vi "0 OCU.vi"(9 "Overview Image Ref In":T11, 10 "Map Name":T3="LPB Pool", 11 "Location of THINK":T14="127.0.0.1") -> ()   [LabVIEW 2011]
doc: "This is the current implementation of the operator control unit (OCU) for sailbot interfacing with this OCU over a network connection. The following features are currently implemented:\n- override control of the rudden angle and sail value by control interface or using keys\n- ability to add missions before and during a run, by clicking and by using GPS location of the boat or an auxiliary GPS attached to the OCU computer\n- modification of tuning values used on the boat\n- indicators for all relevant system status information\n\nAuthors: Jared Kirschner, Jason Curtis"
uses:
  2-Think/2 Typedefs/sail setpt.ctl
  2-Think/2 Typedefs/rudder angle.ctl
  2-Think/2 Typedefs/setpoints to boat.ctl
  0x2-OCU-Think Comm/0x2 Typedefs/manual override.ctl
  2-Think/2 Typedefs/eStopCommand.ctl
  0x2-OCU-Think Comm/0x2 Typedefs/Current Waypoint.ctl
  2-Think/2 Typedefs/UTM Location.ctl
  0x2-OCU-Think Comm/0x2 Classes/NetworkStreams/Reader/NetworkStreamReader.lvclass
  0x2-OCU-Think Comm/0x2 Classes/NetworkStreams/Reader/readType.ctl
  0x2-OCU-Think Comm/0x2 Typedefs/ocuMessage.ctl
  0x2-OCU-Think Comm/0x2 Typedefs/ocuCommands.ctl
  0x2-OCU-Think Comm/0x2 Classes/NetworkStreams/Writer/NetworkStreamWriter.lvclass
  2-Think/2 Typedefs/indicator LED.ctl
  2-Think/2 Typedefs/generalized sensor status.ctl
  2-Think/2 Typedefs/generalized actuator status.ctl
  2-Think/2 Typedefs/Which Boat.ctl
  2-Think/2 Typedefs/robot velocity.ctl
  2-Think/2 Typedefs/heading.ctl
  2-Think/2 Typedefs/rate of turn.ctl
  2-Think/2 Typedefs/pitch and roll.ctl
  2-Think/2 Typedefs/apparent wind.ctl
  2-Think/2 Typedefs/apparent wind speed.ctl
  2-Think/2 Typedefs/apparent wind direction.ctl
  2-Think/2 Typedefs/Velocity.ctl
  2-Think/2 Typedefs/absolute wind direction.ctl
  2-Think/2 Typedefs/absolute wind speed.ctl
  2-Think/2 Typedefs/absolute water current vector.ctl
  0x2-OCU-Think Comm/0x2 Typedefs/RIO-OCU update controls.ctl
  2-Think/2 Classes/Waypoint/Waypoint.lvclass
  0 Typedefs/Mission Type Radio Buttons.ctl
  2-Think/2 Classes/Missions/RoundBuoy/RoundBuoy.lvclass
  2-Think/2 Classes/Missions/PassBuoys/PassBuoys.lvclass
  2-Think/2 Classes/Missions/StationKeeping/StationKeeping.lvclass
  2-Think/2 Classes/Missions/Drive/DriveTo.lvclass
  2-Think/2 Typedefs/Goodness Fns Indicator.ctl
  2-Think/2 Typedefs/UTM Circle.ctl
  2-Think/2 Globals/2 Global.vi
  2-Think/2 Classes/Missions/GenericMission/GenericMission.lvclass
  2-Think/2 Typedefs/tacking attempt.ctl
  0 Typedefs/Sail Position.ctl
  0 Typedefs/Rudder Position.ctl
  0 Typedefs/Apparent Wind Point of Sail.ctl
  0x2-OCU-Think Comm/0x2 Typedefs/ocuWaypoint.ctl
  0x2-OCU-Think Comm/0x2 Typedefs/Waypoints List.ctl
  2-Think/2 Typedefs/PI Constants.ctl
  2-Think/2 Typedefs/Goodness Weightings.ctl
  0 Typedefs/Maps.ctl
  0 Typedefs/Location of Think.ctl
  <vilib>/vision/Image Controls.llb/IMAQ Image.ctl
  2-Think/2 Typedefs/Apparent Wind Mode.ctl
  0x2-OCU-Think Comm/0x2 Typedefs/Sail Setting Tuning.ctl
  0x2-OCU-Think Comm/0x2 Typedefs/Control values.ctl
panel:
  in  "Enable \nLocal GPS":bool
  out "Sensor Status":T1
  in  "GPS COM port":refnum<visa-resource-name>="COM1"
  in  "Additional inputs":T4(tab)
  in  "Manual Mission Input":enum32{"Drive", "Round", "Pass", "Station"}(tab)
  in  "Waypoint Location":enum32{"0", "1", "2", "3", "4"}(radio)
  in  "Buoy Side":enum32{"Starboard", "Port"}(radio)
  in  "Buoy to Round":enum32{"0", "1", "2", "3", "4"}(radio)
  in  "Starboard Buoy":enum32{"0", "1", "2", "3", "4"}(radio)=enum."1"
  in  "Port Buoy":enum32{"0", "1", "2", "3", "4"}(radio)
  in  "Buoy B":enum32{"0", "1", "2", "3", "4"}(radio)=enum."1"
  in  "Buoy A":enum32{"0", "1", "2", "3", "4"}(radio)
  in  "Add Mission":bool
  in  "Stored Locations Array":T5[](array[typedef])=[{"UTM Zone"=0.0, "Hemisphere"=enum."North", "East"=0.0, "North"=0.0}, {"UTM Zone"=0.0, "Hemisphere"=enum."North", "East"=0.0, "North"=0.0}, {"UTM Zone"=0.0, "Hemisphere"=enum."North", "East"=0.0, "North"=0.0}, {"UTM Zone"=0.0, "Hemisphere"=enum."North", "East"=0.0, "North"=0.0}, {"UTM Zone"=0.0, "Hemisphere"=enum."North", "East"=0.0, "North"=0.0}] {"North" format="%#_10f"; "East" format="%#_8f"}
  in  "Boat to Point 0":bool
  in  "Boat to Point 1":bool
  in  "Boat to Point 2":bool
  in  "Boat to Point 3":bool
  in  "Boat to Point 4":bool
  in  "Local to Point 4":bool
  in  "Local to Point 3":bool
  in  "Local to Point 2":bool
  in  "Local to Point 1":bool
  in  "Local to Point 0":bool
  in  "Update Constants":bool
  in  "Tuning Values":T6={"Goodness Weightings"={"Target Importance"=0.8, "No Sail Importance"=1.0, "Change Importance"=0.8, "Pure Waypoint \nImportance"=0.0, "Pure Wind \nImportance"=0.0}, "PI Constants"={"Proportional Gain"=0.5, "Integral Time"=0.0, "Derivative Time"=0.0}, "No Sail Zone\nTuning Quotient"=0.05, "Heading Change Wind Adjustment"=0.2, "Waypoint Tuning Quotient"=10.0, "Apparent Wind Mode"={"Desired Apparent\nWind Direction"=0.0, "On"=FALSE}, "Let Sail Out on Windcross"=TRUE, "Shift Goal for currents"=FALSE, "Round Buoy Safety"=5.0, "Sail Setting Options"={"Linear\nMode"=FALSE, "Sails Full In Point"=85.0, "Sails Full Out Point"=180.0}, "Defilter Wind Data"=TRUE, "Irons Range"=10.0, "Force tack attempt?"=FALSE, "Minimum\ntack try\ntime?"=35.0} {"Sail Setting Options"."Sails Full Out Point" step=0.1; "Sail Setting Options"."Sails Full In Point" step=0.1; "Apparent Wind Mode"."Desired Apparent\nWind Direction" step=0.1; "Goodness Weightings"."Pure Wind \nImportance" min=0.0 step=0.2; "Goodness Weightings"."Pure Waypoint \nImportance" min=0.0 step=0.2; "Goodness Weightings"."Change Importance" min=0.0 step=0.2; "Goodness Weightings"."No Sail Importance" min=0.0 step=0.2; "Goodness Weightings"."Target Importance" min=0.0 step=0.2}
  out "Battery Voltage":dbl
  out "Which Boat Am I?":T12
  out "Rudder Position":T13 scale=50.0..-50.0 scale format="%#.2g"
  out "Connected?":bool caption="Connection Status"
  in  "OVERRIDE SAIL?":bool
  in  "OVERRIDE RUDDER?":bool
  in  "Stop":bool
  in  "OCU Tab Control":enum32{"Mission [M]ap", "Detailed [T]elemetry"}(tab)
  in  "Map Mode":enum32{"M[i]ssion Edit", "M[o]nitoring"}(tab)
  in  "Load MDF":bool
  in  "Time(s)":dbl=300.0
  in  "Tolerance":dbl=3.0
  in  "Mission Entry Type":T15
  in  "Mission Def Filepath":path caption="MDF (Mission Definition File) path"
  in  "Reset Missions/Waypts":bool
  in  "Save Waypoints\nand PoI":bool
  out "Heading":T16 format="%05.1f"
  in  "Plot Colors":T17={"Target"=3381759, "No Sail"=16711680, "Change"=16756736, "Pure Waypt"=35080, "Pure Wind"=16860, "Combined"=16777228}
  out "Goodness Functions":picture
  out "Apparent Wind Direction\nPoint of Sail":T18 scale=0.0..360.0 scale format="%4d"
  out "Mission Status":string caption="Current Mission\nStatus"
  out "Tacking Attempt":T19
  in  "Log message":string caption="Log message (type and press enter)"
  in  "Save Image":bool
  out "Mission Map":T11(plugin-control)
  in  "Overlay Font Size":i16=40
  out "# of Waypts":i32
  in  "Globals":T20(tab)
  out "Don't Tip?":bool
  out "Wind Sensor Status":T1
  out "Estimated Error":dbl
  out "Robot Heading":T16 format="%05.1f"
  out "Robot UTM Location":T5 {"North" format="%#_10f"; "East" format="%#_8f"}
  out "Robot Velocity":T21
  out "Robot\nRate of Turn":T22 format="%05.1f"
  out "Robot Pitch/Roll":T23 {"Roll" format="%05.1f"; "Pitch" format="%05.1f"}
  out "Robot Speed (m/s)":dbl
  out "Absolute Wind":T24 {"East" format="%#_5g"}
  out "Apparent Wind Direction":T25
  out "Apparent Wind Speed":T26
  out "Apparent Wind":T27
  out "Crossing Wind":bool
  out "Setpoints to boat":T28
  out "Sail Position":T29
  out "Rudder Angle":T30
  out "Current Waypoint":T31
  in  "Reset to start":bool
  out "Manual Override":T32
  out "Waypoints Array":T33[](array[typedef]) {"UTM Location"."North" format="%#_10f"; "UTM Location"."East" format="%#_8f"}
  out "Waypoints Object Array":T34
  out "Mission Object Array":refnum<class "GenericMission.lvclass">[](array[class])
  out "Global No Sail Circles":T35[](array[typedef])
  out "Sail Position":T36
  # "PORT"
  # "STARB"
  # "Local GPS"
  # "Note: if THINK\nis on this computer,\nturning on local GPS will do strange things."
  # "HOWTO:\n1. save one or more points by moving GPS sensor to point, and pressing buttons below\n2. choose type of mission from tab control\n3. choose saved point(s) to load into mission. other params come from mission map input above\n4. click \"Add Mission\""
  # "P"
  # "S"
  # "O"
  # "O"
  # "A"
  # "B"
  # "HOWTO:\nchange values here, \nthen hit:"
  # "inputting missions:\nGo To Waypoint: set tolerance, and click on map.\nRound Buoy Port/Starboard: set tolerance, click.\nPass Between Buoys: Click one buoy location\nand drag to the other.\nStation Keeping: click southwest corner, drag to \nsoutheast corner. A square will be generated.\nTime(s) currently unimplemented.\nGlobal No-Sail Zone: click center of zone, drag to edge of\nzone. A circle with appropriate radius will be created."
  # "As Measured"
  # "Path Planning"
  # "From Planning Functions"
  # "(this is not a cluster because subitems\nare generated in parallel code)"
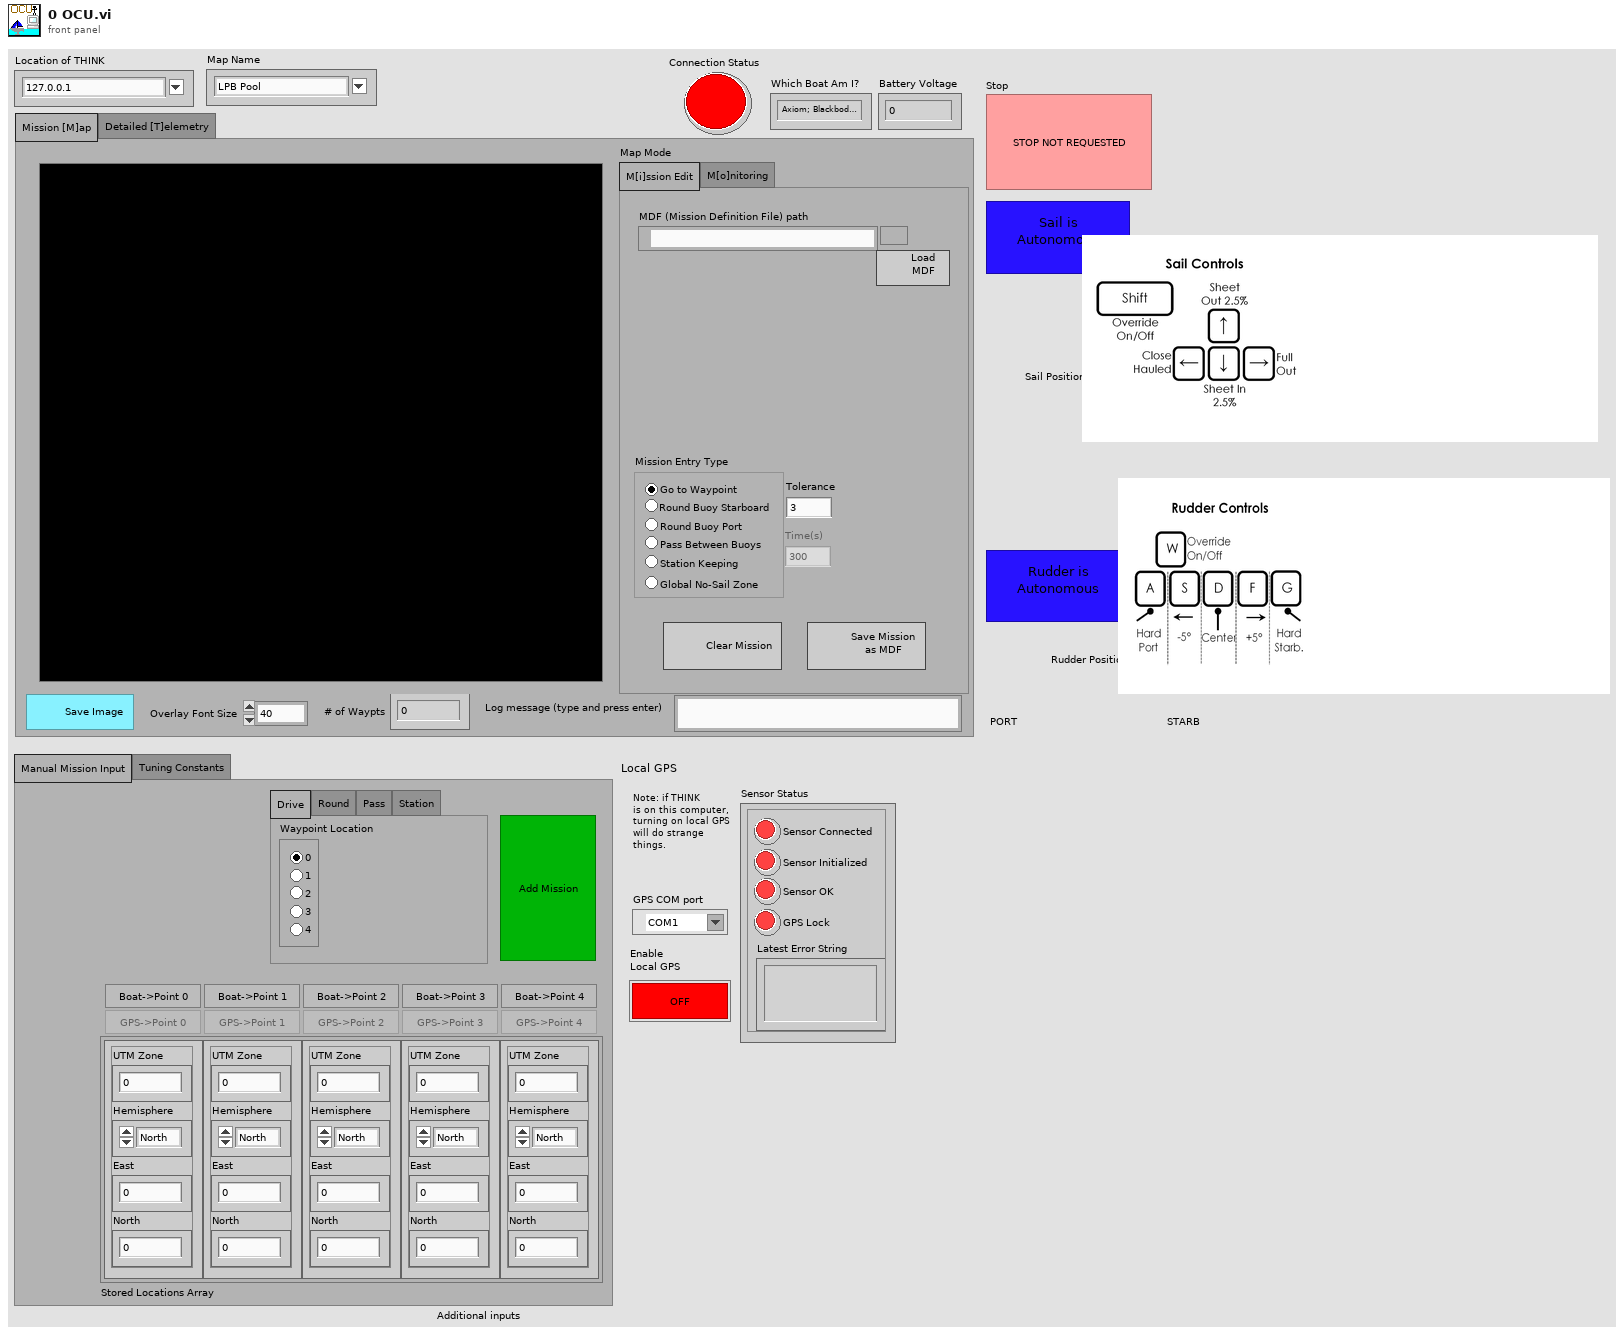
[diagram p1: front panel]
types:
  T1 = typedef "generalized sensor status.ctl" = cluster{"Sensor Connected":T2, "Sensor Initialized":T2, "Sensor OK":T2, "Latest Error String":string, "GPS Lock":T2}
  T2 = typedef "indicator LED.ctl" = bool
  T3 = typedef "Maps.ctl" = string
  T4 = enum32{"Manual Mission Input", "Tuning Constants"}
  T5 = typedef "UTM Location.ctl" = cluster{"UTM Zone":dbl, "Hemisphere":enum16{"North", "South"}, "East":dbl, "North":dbl}
  T6 = typedef "Control values.ctl" = cluster{"Goodness Weightings":T7, "PI Constants":T8, "No Sail Zone\nTuning Quotient":dbl, "Heading Change Wind Adjustment":dbl, "Waypoint Tuning Quotient":dbl, "Apparent Wind Mode":T9, "Let Sail Out on Windcross":bool, "Shift Goal for currents":bool, "Round Buoy Safety":dbl, "Sail Setting Options":T10, "Defilter Wind Data":bool, "Irons Range":dbl, "Force tack attempt?":bool, "Minimum\ntack try\ntime?":dbl}
  T7 = typedef "Goodness Weightings.ctl" = cluster{"Target Importance":dbl, "No Sail Importance":dbl, "Change Importance":dbl, "Pure Waypoint \nImportance":dbl, "Pure Wind \nImportance":dbl}
  T8 = typedef "PI Constants.ctl" = cluster{"Proportional Gain":dbl, "Integral Time":dbl, "Derivative Time":dbl}
  T9 = typedef "Apparent Wind Mode.ctl" = cluster{"Desired Apparent\nWind Direction":dbl, "On":bool}
  T10 = typedef "Sail Setting Tuning.ctl" = cluster{"Linear\nMode":bool, "Sails Full In Point":dbl, "Sails Full Out Point":dbl}
  T11 = typedef "IMAQ Image.ctl" = refnum<image>
  T12 = typedef "Which Boat.ctl" = enum16{"Axiom; Blackbody Radiation", "Simulation"}
  T13 = typedef "Rudder Position.ctl" = dbl
  T14 = typedef "Location of Think.ctl" = string
  T15 = typedef "Mission Type Radio Buttons.ctl" = enum32{"Go to Waypoint", "Round Buoy Starboard", "Round Buoy Port", "Pass Between Buoys", "Station Keeping", "Global No-Sail Zone"}
  T16 = typedef "heading.ctl" = dbl
  T17 = cluster{"Target":u32, "No Sail":u32, "Change":u32, "Pure Waypt":u32, "Pure Wind":u32, "Combined":u32}
  T18 = typedef "Apparent Wind Point of Sail.ctl" = dbl
  T19 = typedef "tacking attempt.ctl" = cluster{"attempting tack":bool, "tacking attempt\ntime remaining":dbl}
  T20 = enum32{"How Am I", "Where Am I", "What's Around Me", "Path Planning"}
  T21 = typedef "robot velocity.ctl" = cluster{"East":dbl, "North":dbl}
  T22 = typedef "rate of turn.ctl" = dbl
  T23 = typedef "pitch and roll.ctl" = cluster{"Pitch":dbl, "Roll":dbl}
  T24 = typedef "Velocity.ctl" = cluster{"East":dbl, "North":dbl}
  T25 = typedef "apparent wind direction.ctl" = dbl
  T26 = typedef "apparent wind speed.ctl" = dbl
  T27 = typedef "apparent wind.ctl" = cluster{"Toward Fore":dbl, "Toward Starboard":dbl}
  T28 = typedef "setpoints to boat.ctl" = cluster{"Sail Position":T29, "Rudder Angle":T30}
  T29 = typedef "sail setpt.ctl" = dbl
  T30 = typedef "rudder angle.ctl" = dbl
  T31 = typedef "Current Waypoint.ctl" = i32
  T32 = typedef "manual override.ctl" = cluster{"Override Active Rudder":bool, "Setpoints":T28, "Override Active Sail":bool}
  T33 = typedef "ocuWaypoint.ctl" = cluster{"Tolerance (m)":dbl, "UTM Location":T5}
  T34 = typedef "Waypoints List.ctl" = refnum<class "Waypoint.lvclass">[]
  T35 = typedef "UTM Circle.ctl" = cluster{"UTM Zone":dbl, "Hemisphere":enum16{"North", "South"}, "East":dbl, "North":dbl, "Radius":dbl}
  T36 = typedef "Sail Position.ctl" = dbl
  T37 = typedef "RIO-OCU update controls.ctl" = cluster{"Sensor Status":T1, "Battery Voltage":dbl, "Rudder Actuator Status":T38, "Sail Actuator Status":T38, "Which Boat Am I?":T12, "Robot Velocity":T21, "Robot UTM Location":T5, "Robot\nHeading ":T16, "Robot\nRate of Turn":T22, "Robot Pitch/Roll":T23, "Apparent Wind":T27, "Apparent Wind\nSpeed":T26, "Apparent Wind\nDirection (º)":T25, "Absolute Wind":T24, "Absolute Wind\nDirection (º)":T39, "Absolute Wind\nSpeed":T40, "Absolute Water Current Vector":T41, "Rudder Angle":T30, "Sail Position":T29, "Manual Override Cluster":T32, "Setpoints to boat":T28, "Current Waypoint":T31, "Think freq.":dbl, "Sense freq.":dbl, "Act freq.":dbl, "E-stop freq.":dbl, "Network \nfreq.":dbl, "Network \nLoop Iterations":i64, "E-Stop":bool, "Serialized Waypoint Array":string, "Serialized Mission Queue Elements":string, "Goodness Functions":T42, "Global No Sail Circles":T35[], "Optimal Heading":dbl, "Crossing Wind":bool, "Estimated Error":dbl, "Don't Tip?":bool, "Tacking Attempt":T19}
  T38 = typedef "generalized actuator status.ctl" = cluster{"Actuator Connected":T2}
  T39 = typedef "absolute wind direction.ctl" = dbl
  T40 = typedef "absolute wind speed.ctl" = dbl
  T41 = typedef "absolute water current vector.ctl" = cluster{"Direction":T25, "Magnitude":T25}
  T42 = typedef "Goodness Fns Indicator.ctl" = cluster{dbl, dbl, dbl[][]}
  T43 = typedef "0-Image Descriptor.ctl" = cluster{"Upper-Left Corner Coordinates":T5, "Meters/Pixel":dbl}
  T44 = typedef "NetworkStreamReader.lvclass/readType.ctl" = enum16{"Next in buffer", "Most current"}
  T45 = typedef "eStopCommand.ctl" = enum16{"Reset E-Stop", "Get E-Stop", "Set E-Stop"}
  T46 = cluster{"Image Ref Out":T11, "Image Descriptor":T43}
  T47 = typedef "ocuMessage.ctl" = cluster{"OCU Command":T48, "Data":variant}
  T48 = typedef "ocuCommands.ctl" = enum16{"Pass", "Send override", "Set waypoint number", "Stop", "Add Mission", "Reset Missions/Waypts", "Edit Control Values", "Add Global No-Sail", "Log Message"}
  T49 = enum8{"Enabled", "Disabled", "Disabled and Grayed Out"}
  T50 = typedef "eventvkey.ctl" = enum16{"ASCII", "Enter", "Return", "Shift", "Ctrl", "Alt", "Cmd", "Opt", "Caps", "NumLock", "Clear", "Break", "Up", "Down", "Left", "Right", "Insert", "Delete", "Home", "End", "PageUp", "PageDown", "Escape", "Help", "Pause", "ScrollLock", "F1", "F2", "F3", "F4", "F5", "F6", "F7", "F8", "F9", "F10", "F11", "F12", "F13", "F14", "F15", "F16", "F17", "F18", "F19", "F20", "F21", "F22", "F23", "F24", "Play", "VolumeUp", "VolumeDown", "Mute", "Two Byte Char"}
  T51 = cluster{"Global Rectangle":i32[], "Contours":cluster{"Contour Type":u32, "ROI Type":u32, "Points":i32[]}[]}
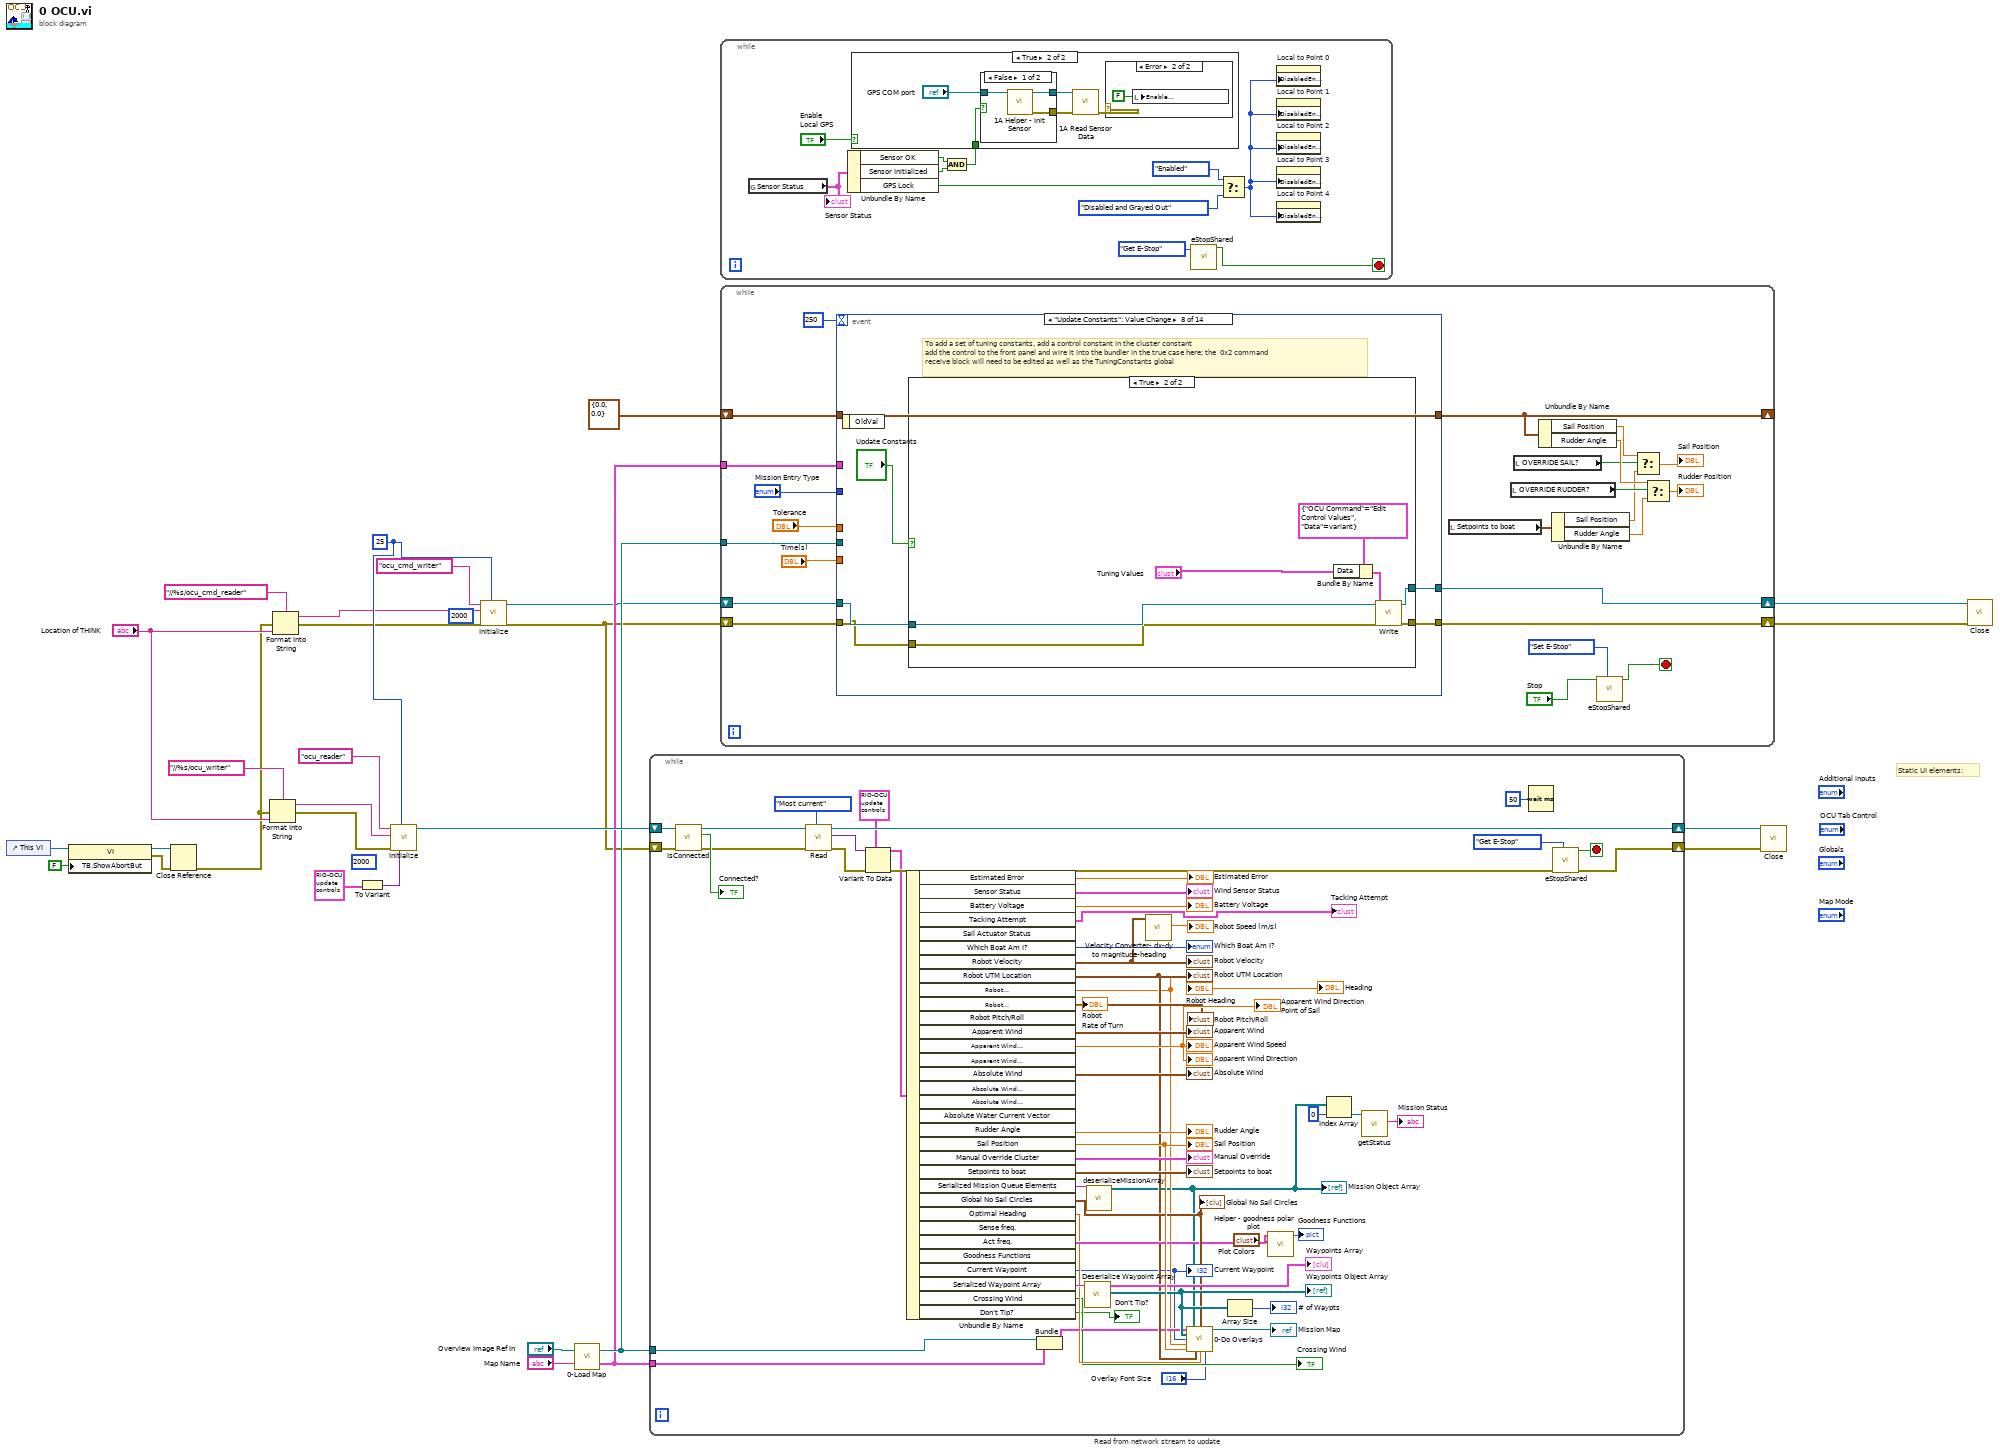
[diagram p0: block diagram]
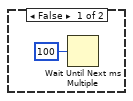
[diagram p2: hidden frame]
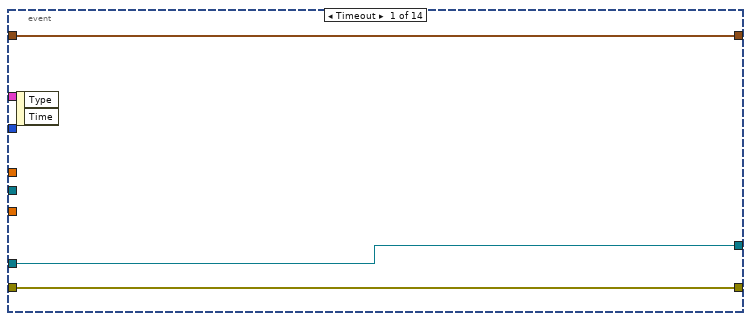
[diagram p5: hidden frame]
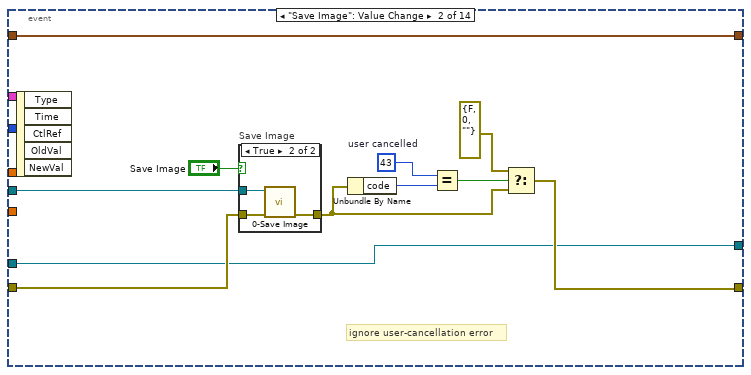
[diagram p6: hidden frame]
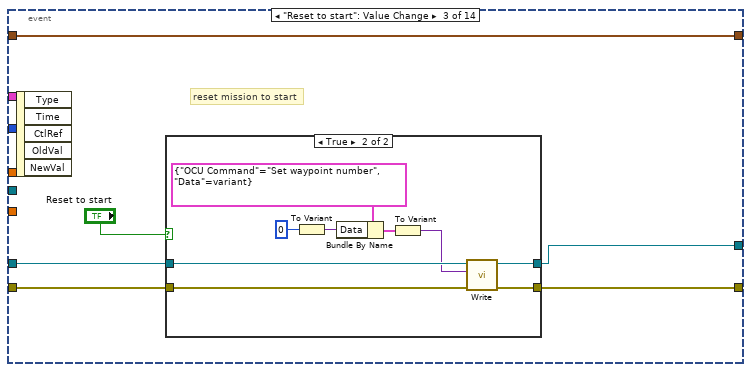
[diagram p8: hidden frame]
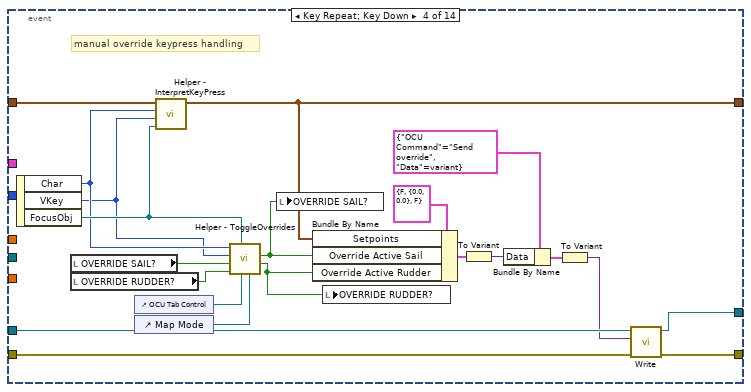
[diagram p10: hidden frame]
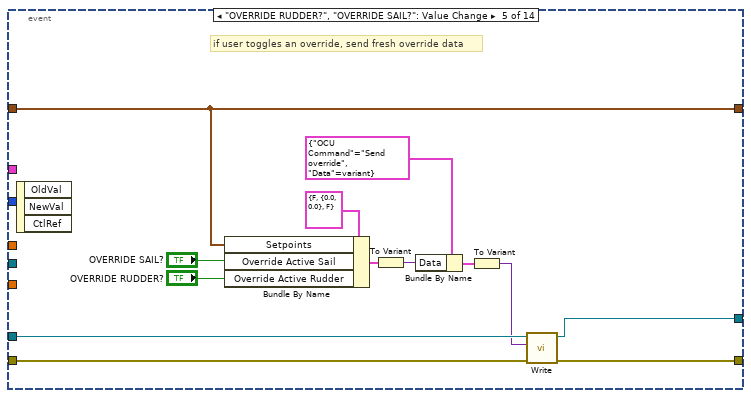
[diagram p11: hidden frame]
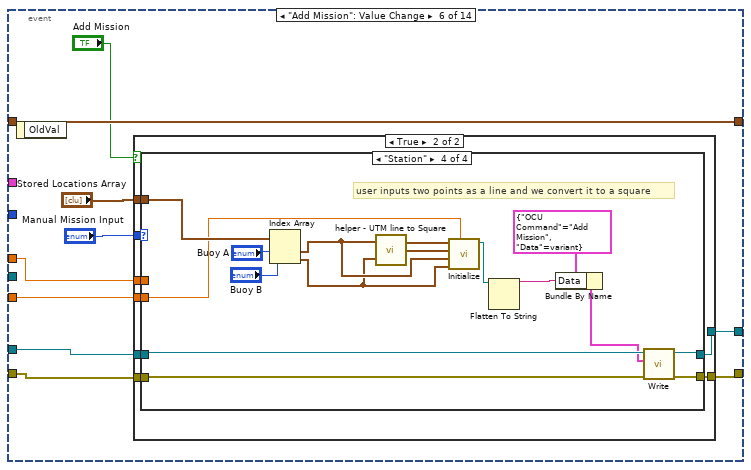
[diagram p12: hidden frame]
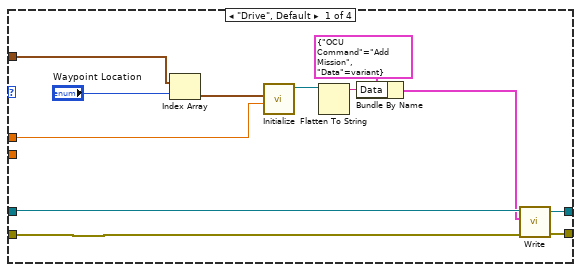
[diagram p14: hidden frame]
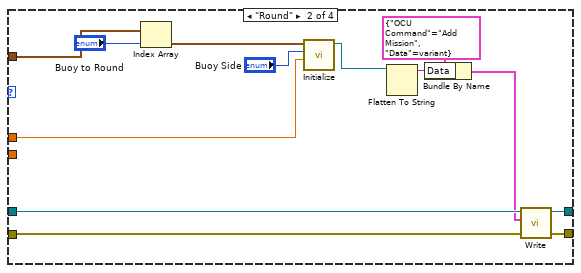
[diagram p15: hidden frame]
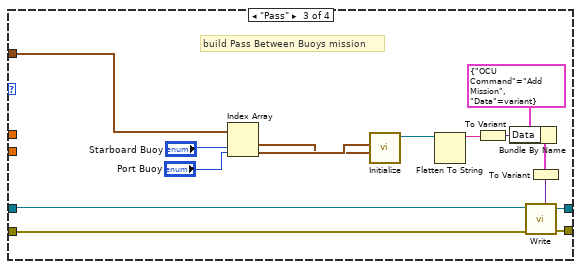
[diagram p16: hidden frame]
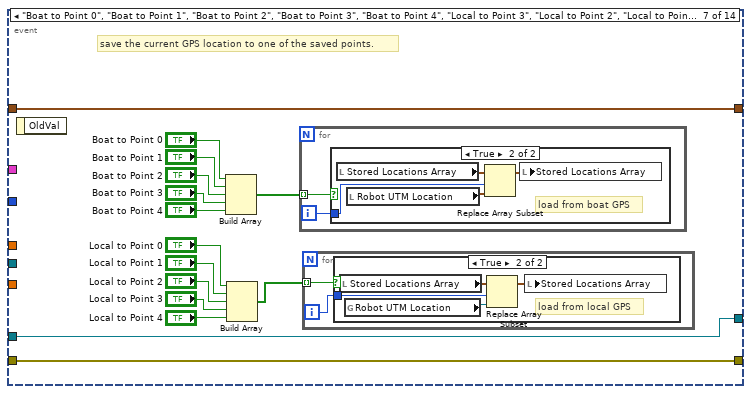
[diagram p17: hidden frame]
diagram:
  (unwired) 2000 ("connection timeout")
  (unwired) 2000 ("connection timeout")
  w27 = 25 ("writer buffer size")
  # "Static UI elements:"
  n1 = control-ref of="This VI"() -> (w17:refnum<vi>)
  n2 = property class="VI"(reference=w17, "TB.ShowAbortBut"=FALSE ("Tool Bar:Show Abort Button")) -> (reference out=w15:refnum<vi>, error out=w14:errorcluster)  [unwired: 1 in]
  n3 = Close Reference(reference=w15, error in (no error)=w14) -> (error out=w13:errorcluster)
  n4 = Format Into String(format string="//%s/ocu_writer", error in=w13, "Location of THINK") -> (resulting string=w7:string, error out=w11:errorcluster)  [unwired: 1 in]
  n5 = Format Into String(format string="//%s/ocu_cmd_reader", error in=w13, "Location of THINK") -> (resulting string=w5:string, error out=w12:errorcluster)  [unwired: 1 in]
  n6 = To Variant(anything=T37 {"Sensor Status"={"Sensor Connected"=FALSE, "Sensor Initialized"=FALSE, "Sensor OK"=FALSE, "Latest Error String"="", "GPS Lock"=FALSE}, "Battery Voltage"=0.0, "Rudder Actuator Status"={"Actuator Connected"=FALSE}, "Sail Actuator Status"={"Actuator Connected"=FALSE}, "Which Boat Am I?"=enum."Axiom; Blackbody Radiation", "Robot Velocity"={"East"=0.0, "North"=0.0}, "Robot UTM Location"={"UTM Zone"=0.0, "Hemisphere"=enum."North", "East"=0.0, "North"=0.0}, "Robot\nHeading "=0.0, "Robot\nRate of Turn"=0.0, "Robot Pitch/Roll"={"Pitch"=0.0, "Roll"=0.0}, "Apparent Wind"={"Toward Fore"=0.0, "Toward Starboard"=0.0}, "Apparent Wind\nSpeed"=0.0, "Apparent Wind\nDirection (º)"=0.0, "Absolute Wind"={"East"=0.0, "North"=0.0}, "Absolute Wind\nDirection (º)"=0.0, "Absolute Wind\nSpeed"=0.0, "Absolute Water Current Vector"={"Direction"=0.0, "Magnitude"=0.0}, "Rudder Angle"=0.0, "Sail Position"=0.0, "Manual Override Cluster"={"Override Active Rudder"=FALSE, "Setpoints"={"Sail Position"=0.0, "Rudder Angle"=0.0}, "Override Active Sail"=FALSE}, "Setpoints to boat"={"Sail Position"=0.0, "Rudder Angle"=0.0}, "Current Waypoint"=0, "Think freq."=0.0, "Sense freq."=0.0, "Act freq."=0.0, "E-stop freq."=0.0, "Network \nfreq."=0.0, "Network \nLoop Iterations"=0, "E-Stop"=FALSE, "Serialized Waypoint Array"="", "Serialized Mission Queue Elements"="", "Goodness Functions"={0.0, 0.0, []}, "Global No Sail Circles"=[], "Optimal Heading"=0.0, "Crossing Wind"=FALSE, "Estimated Error"=0.0, "Don't Tip?"=FALSE, "Tacking Attempt"={"attempting tack"=FALSE, "tacking attempt\ntime remaining"=0.0}} ("RIO->OCU update data")) -> (Variant=w26:variant)
  n7 = call "Initialize.vi"("Default return"=w26, "reader buffer size"=w27, "error in (no error)"=w11, "writer url"=w7, "reader name"="ocu_reader" ("writer name")) -> ("NetworkStreamWriter out"=w28:refnum<class "NetworkStreamReader.lvclass">)  [unwired: 5 in, 1 out]
  n8 = call "Initialize.vi"("writer buffer size"=w27, "error in (no error)"=w12, "reader url"=w5, "writer name"="ocu_cmd_writer") -> ("error out"=w1:errorcluster, "NetworkStreamWriter out"=w2:refnum<class "NetworkStreamWriter.lvclass">)  [unwired: 6 in]
  n9 = call "0-Load Map.vi"("Map Name"="Map Name", "Image Ref In"="Overview Image Ref In") -> ("Image Descriptor"=w9:T43, "Image Ref Out"=w23:T11)
  n10 = while "Read from network stream to update" {
    shift-right: [w86] -> w25
    shift-left: w28 -> [w81]
    shift-right: [w79] -> w24
    shift-left: w1 -> [w80]
    tunnel: w23 -> [w83]
    tunnel: w9 -> [w82]
    stop <- w84 stop-if-true
    n11 = call "IsConnected.vi"("error in (no error)"=w80, "NetworkStreamReader in"=w81) -> ("error out"=w75:errorcluster, "Connected?"=→"Connected?":bool, "NetworkStreamReader out"=w76:refnum<class "NetworkStreamReader.lvclass">)  [unwired: 7 in]
    n12 = call "Read.vi"("Read Type"=readType."Most current", "error in (no error)"=w75, "NetworkStreamReader in"=w76) -> ("error out"=w72:errorcluster, "element"=w71:variant, "NetworkStreamReader out"=w86:refnum<class "NetworkStreamReader.lvclass">)  [unwired: 4 in, 2 out]
    n13 = Variant To Data(error in=w72, type=T37 {"Sensor Status"={"Sensor Connected"=FALSE, "Sensor Initialized"=FALSE, "Sensor OK"=FALSE, "Latest Error String"="", "GPS Lock"=FALSE}, "Battery Voltage"=0.0, "Rudder Actuator Status"={"Actuator Connected"=FALSE}, "Sail Actuator Status"={"Actuator Connected"=FALSE}, "Which Boat Am I?"=enum."Axiom; Blackbody Radiation", "Robot Velocity"={"East"=0.0, "North"=0.0}, "Robot UTM Location"={"UTM Zone"=0.0, "Hemisphere"=enum."North", "East"=0.0, "North"=0.0}, "Robot\nHeading "=0.0, "Robot\nRate of Turn"=0.0, "Robot Pitch/Roll"={"Pitch"=0.0, "Roll"=0.0}, "Apparent Wind"={"Toward Fore"=0.0, "Toward Starboard"=0.0}, "Apparent Wind\nSpeed"=0.0, "Apparent Wind\nDirection (º)"=0.0, "Absolute Wind"={"East"=0.0, "North"=0.0}, "Absolute Wind\nDirection (º)"=0.0, "Absolute Wind\nSpeed"=0.0, "Absolute Water Current Vector"={"Direction"=0.0, "Magnitude"=0.0}, "Rudder Angle"=0.0, "Sail Position"=0.0, "Manual Override Cluster"={"Override Active Rudder"=FALSE, "Setpoints"={"Sail Position"=0.0, "Rudder Angle"=0.0}, "Override Active Sail"=FALSE}, "Setpoints to boat"={"Sail Position"=0.0, "Rudder Angle"=0.0}, "Current Waypoint"=0, "Think freq."=0.0, "Sense freq."=0.0, "Act freq."=0.0, "E-stop freq."=0.0, "Network \nfreq."=0.0, "Network \nLoop Iterations"=0, "E-Stop"=FALSE, "Serialized Waypoint Array"="", "Serialized Mission Queue Elements"="", "Goodness Functions"={0.0, 0.0, []}, "Global No Sail Circles"=[], "Optimal Heading"=0.0, "Crossing Wind"=FALSE, "Estimated Error"=0.0, "Don't Tip?"=FALSE, "Tacking Attempt"={"attempting tack"=FALSE, "tacking attempt\ntime remaining"=0.0}} ("RIO->OCU update data"), Variant=w71) -> (data=w69:T37, error out=w74:errorcluster)
    n14 = Unbundle By Name(w69) -> ("Estimated Error"=→"Estimated Error":dbl, "Sensor Status"=→"Wind Sensor Status":T1, "Battery Voltage"=→"Battery Voltage":dbl, "Tacking Attempt"=→"Tacking Attempt":T19, "Which Boat Am I?"=→"Which Boat Am I?":T12, "Robot Velocity"=w33:T21, "Robot UTM Location"=w45:T5, "Robot\nHeading"=w41:T16, "Robot\nRate of Turn"=→"Robot\nRate of Turn":T22, "Robot Pitch/Roll"=→"Robot Pitch/Roll":T23, "Apparent Wind"=→"Apparent Wind":T27, "Apparent Wind\nSpeed"=→"Apparent Wind Speed":T26, "Apparent Wind\nDirection (º)"=→"Apparent Wind Direction" →"Apparent Wind Direction\nPoint of Sail":T25, "Absolute Wind"=→"Absolute Wind":T24, "Rudder Angle"=→"Rudder Angle":T30, "Sail Position"=w57:T29, "Manual Override Cluster"=→"Manual Override":T32, "Setpoints to boat"=→"Setpoints to boat":T28, "Serialized Mission Queue Elements"=w52:string, "Global No Sail Circles"=w49:T35[], "Optimal Heading"=w44:dbl, "Goodness Functions"=w48:T42, "Current Waypoint"=w35:T31, "Serialized Waypoint Array"=w56:string, "Crossing Wind"=→"Crossing Wind":bool, "Don't Tip?"=→"Don't Tip?":bool)  [unwired: 6 out]
    "Robot UTM Location" <- w45
    "Robot Heading" <- w41
    "Robot Velocity" <- w33
    "Sail Position" <- w57
    "Current Waypoint" <- w35
    "Global No Sail Circles" <- w49
    "Heading" <- w41
    n15 = Bundle("Image Ref Out"=w83, "Image Descriptor"=w82) -> (w43:T46)  [unwired: 1 in]
    n16 = call "Deserialize Waypoint Array.vi"("Serialized Waypoint Array"=w56) -> ("Waypoints Object Array"=w54:T34, "Waypoints Array"=→"Waypoints Array":T33[])  [unwired: 9 in]
    "Waypoints Object Array" <- w54
    n17 = call "deserializeMissionArray.vi"("Serialized Mission Array"=w52) -> ("Mission Object Array"=w36:refnum<class "GenericMission.lvclass">[])  [unwired: 9 in, 1 out]
    "Mission Object Array" <- w36
    n18 = call "Velocity Converter- dx-dy to magnitude-heading.vi"("Vector In"=w33) -> ("Magnitude Out"=→"Robot Speed (m/s)":dbl)  [unwired: 9 in, 1 out]
    n19 = call "0-Do Overlays.vi"("Image Reference\nand Descriptor"=w43, "Missions"=w36, "No Sail Circles"=w49, "Waypoints"=w54, "Current Waypoint #"=w35, "Heading"=w41, "Sail Position"=w57, "Robot UTM Location"=w45, "Optimal Heading"=w44, "Font Size"="Overlay Font Size") -> ("Image out"=→"Mission Map":T11)  [unwired: 5 in]
    n20 = Array Size(array=w54) -> (size(s)=→"# of Waypts":i32)
    n21 = call "Helper - goodness polar plot.vi"("Plot Colors"="Plot Colors", "Goodness Fns In"=w48) -> ("Goodness Functions Polar Plot"=→"Goodness Functions":picture)  [unwired: 9 in]
    n22 = Index Array(array=w36, index=0) -> (element=w37:refnum<class "GenericMission.lvclass">)
    n23 = call-dynamic "getStatus.vi"("GenericMission in"=w37) -> ("Status"=→"Mission Status":string)  [unwired: 8 in, 2 out]
    n24 = Wait (ms)(milliseconds to wait=u32 50 ("millisecond multiple")) -> ()  [unwired: 1 out]
    n25 = call "eStopShared.vi"("Command"=eStopCommand."Get E-Stop", "Error In"=w74) -> ("Error Out"=w79:errorcluster, "E-Stop Out"=w84:bool)  [unwired: 8 in]
  }
  n26 = while {
    shift-right: [w108] -> w18
    shift-left: w1 -> [w87]
    shift-right: [w102] -> _
    shift-left: T28 {"Sail Position"=0.0, "Rudder Angle"=0.0} ("Setpoints") -> [w110]
    shift-right: [w104] -> w19
    shift-left: w2 -> [w88]
    tunnel: w23 -> [w103]
    tunnel: w9 -> [w101]
    stop <- w107 stop-if-true
    n27 = event shown="[7] \"Update Constants\": Value Change" {
      selector: _ -> [_ _ _ _ _ _ _ _ _ _ _ _ _ _]
      dyn-events: _ -> [_ _ _ _ _ _ _ _ _ _ _ _ _ _]
      timeout: 250 -> [_ _ _ _ _ _ _ _ _ _ _ _ _ _]
      tunnel: w110 -> [w113 w120 w134 w166 w169 w187 w263 w287 w309 w325 w334 w375 w393 w513]
      tunnel: [w113 w120 w134 w164 w169 w187 w263 w287 w309 w325 w334 w375 w393 w513] -> w102
      tunnel: w87 -> [w111 w118 w131 w161 w176 w188 w261 w284 w301 w324 w332 w373 w392 w514]
      tunnel: [w111 w115 w129 w160 w175 w185 w261 w282 w299 w324 w331 w371 w390 w514] -> w108
      tunnel: w88 -> [w112 w114 w132 w163 w178 w189 w262 w285 w300 w323 w330 w374 w388 w515]
      tunnel: [w112 w114 w130 w162 w177 w184 w262 w283 w302 w323 w329 w372 w389 w515] -> w104
      tunnel: w103 -> [_ w119 _ _ _ _ _ _ _ _ _ _ _ _]
      tunnel: w101 -> [_ _ _ _ _ _ _ _ _ _ _ _ w391 _]
      tunnel: "Mission Entry Type" -> [_ _ _ _ _ _ _ _ _ _ _ _ w387 _]
      tunnel: "Tolerance" -> [_ _ _ _ _ w186 _ _ _ _ _ _ w386 _]
      tunnel: "Time(s)" -> [_ _ _ _ _ w180 _ _ _ _ _ _ w385 _]
      event Timeout {
        n28 = event-data() -> ()  [unwired: 1 in, 2 out]
      }
      event "Save Image": Value Change {
        w123 = 43  # user cancelled
        # "ignore user-cancellation error"
        n29 = event-data() -> ()  [unwired: 1 in, 5 out]
        n30 = case "Save Image" shown="True" "Save Image" {
          tunnel: w118 -> [w125 w128]
          tunnel: [w125 w127] -> w117
          tunnel: w119 -> [_ w126]
          frame False {
          }
          frame True {
            n31 = call "0-Save Image.vi"("Error In"=w128, "Image in"=w126) -> ("Error Out"=w127:errorcluster)  [unwired: 9 in]
          }
        }
        n32 = Unbundle By Name(w117) -> ("code"=w124:i32)
        n33 = Equal?(x=w123, y=w124) -> (x = y?=w122:bool)
        n34 = Select(t=errorcluster {"status"=FALSE, "code"=0, "source"=""}, s=w122, f=w117) -> (s? t:f=w115:errorcluster)
      }
      event "Reset to start": Value Change {
        # "reset mission to start"
        n35 = event-data() -> ()  [unwired: 1 in, 5 out]
        n36 = case shown="True" "Reset to start" {
          tunnel: w132 -> [w136 w142]
          tunnel: w131 -> [w135 w143]
          tunnel: [w136 w145] -> w130
          tunnel: [w135 w144] -> w129
          frame False {
          }
          frame True {
            n37 = To Variant(anything=T31 0 ("Current Waypoint")) -> (Variant=w140:variant)
            n38 = Bundle By Name(cluster=T47 {"OCU Command"=enum."Set waypoint number", "Data"=variant}, "Data"=w140) -> (w138:T47)
            n39 = To Variant(anything=w138) -> (Variant=w137:variant)
            n40 = call "Write.vi"("error in (no error)"=w143, "element"=w137, "NetworkStreamWriter in"=w142) -> ("error out"=w144:errorcluster, "NetworkStreamWriter out"=w145:refnum<class "NetworkStreamWriter.lvclass">)  [unwired: 7 in]
          }
        }
      }
      event Key Repeat; Key Down {
        # "manual override keypress handling"
        n41 = event-data() -> ("Char"=w153:i16, "VKey"=w152:T50, "FocusObj"=w154:refnum<vi>)  [unwired: 1 in]
        n42 = local read "OVERRIDE SAIL?"() -> (w151:bool)
        n43 = local read "OVERRIDE RUDDER?"() -> (w150:bool)
        n44 = control-ref of="OCU Tab Control"() -> (w147:refnum<vi>)
        n45 = control-ref of="Map Mode"() -> (w146:refnum<vi>)
        n46 = call "Helper - InterpretKeyPress.vi"("FocusObj"=w154, "VKey"=w152, "Char"=w153, "Command In"=w166) -> ("Command Out"=w164:T28)  [unwired: 7 in]
        n47 = call "Helper - ToggleOverrides.vi"("Map Mode Tab Control Ref"=w146, "OCU Tab Control Ref"=w147, "FocusObj"=w154, "Rudder Override?"=w150, "Sail Override?"=w151, "VKey"=w152, "Char"=w153) -> ("Override Rudder"=w149:bool, "Override Sail"=w148:bool)  [unwired: 3 in]
        n48 = local write "OVERRIDE SAIL?"(w148) -> ()
        n49 = Bundle By Name(cluster=T32 {"Override Active Rudder"=FALSE, "Setpoints"={"Sail Position"=0.0, "Rudder Angle"=0.0}, "Override Active Sail"=FALSE} ("Manual Override Cluster"), "Setpoints"=w164, "Override Active Sail"=w148, "Override Active Rudder"=w149) -> (w156:T32)
        n50 = local write "OVERRIDE RUDDER?"(w149) -> ()
        n51 = To Variant(anything=w156) -> (Variant=w159:variant)
        n52 = Bundle By Name(cluster=T47 {"OCU Command"=enum."Send override", "Data"=variant}, "Data"=w159) -> (w158:T47)
        n53 = To Variant(anything=w158) -> (Variant=w155:variant)
        n54 = call "Write.vi"("error in (no error)"=w161, "element"=w155, "NetworkStreamWriter in"=w163) -> ("error out"=w160:errorcluster, "NetworkStreamWriter out"=w162:refnum<class "NetworkStreamWriter.lvclass">)  [unwired: 7 in]
      }
      event "OVERRIDE RUDDER?", "OVERRIDE SAIL?": Value Change {
        # "if user toggles an override, send fresh override data"
        n55 = event-data() -> ()  [unwired: 1 in, 3 out]
        n56 = Bundle By Name(cluster=T32 {"Override Active Rudder"=FALSE, "Setpoints"={"Sail Position"=0.0, "Rudder Angle"=0.0}, "Override Active Sail"=FALSE} ("Manual Override Cluster"), "Setpoints"=w169, "Override Active Sail"="OVERRIDE SAIL?", "Override Active Rudder"="OVERRIDE RUDDER?") -> (w171:T32)
        n57 = To Variant(anything=w171) -> (Variant=w174:variant)
        n58 = Bundle By Name(cluster=T47 {"OCU Command"=enum."Send override", "Data"=variant}, "Data"=w174) -> (w173:T47)
        n59 = To Variant(anything=w173) -> (Variant=w170:variant)
        n60 = call "Write.vi"("error in (no error)"=w176, "element"=w170, "NetworkStreamWriter in"=w178) -> ("error out"=w175:errorcluster, "NetworkStreamWriter out"=w177:refnum<class "NetworkStreamWriter.lvclass">)  [unwired: 7 in]
      }
      event "Add Mission": Value Change {
        n61 = event-data() -> ()  [unwired: 1 in, 1 out]
        n62 = case shown="True" "Add Mission" {
          tunnel: w189 -> [w191 w199]
          tunnel: w188 -> [w190 w198]
          tunnel: w186 -> [_ w197]
          tunnel: [w190 w196] -> w185
          tunnel: [w191 w195] -> w184
          tunnel: "Manual Mission Input" -> [_ w194]
          tunnel: "Stored Locations Array" -> [_ w193]
          tunnel: w180 -> [_ w192]
          frame False {
          }
          frame True {
            n63 = case shown="\"Station\"" w194 {
              tunnel: w198 -> [w207 w220 w229 w247]
              tunnel: [w211 w220 w232 w252] -> w196
              tunnel: w197 -> [w208 w223 _ _]
              tunnel: [w210 w222 w233 w253] -> w195
              tunnel: w199 -> [w209 w221 w234 w251]
              tunnel: w193 -> [w202 w218 w228 w246]
              tunnel: w192 -> [_ _ _ w239]
              frame "Drive", Default {
                n64 = Index Array(array=w202, index="Waypoint Location") -> (element=w205:T5)
                n65 = call "Initialize.vi"("Tolerance (m)"=w208, "Drive Location"=w205) -> ("Drive out"=w203:refnum<class "DriveTo.lvclass">)  [unwired: 8 in, 1 out]
                n66 = Flatten To String(anything=w203) -> (data string=w201:string)  [unwired: 3 in, 2 out]
                n67 = Bundle By Name(cluster=T47 {"OCU Command"=enum."Add Mission", "Data"=variant}, "Data"=w201) -> (w200:T47)
                n68 = call "Write.vi"("error in (no error)"=w207, "element"=w200, "NetworkStreamWriter in"=w209) -> ("error out"=w211:errorcluster, "NetworkStreamWriter out"=w210:refnum<class "NetworkStreamWriter.lvclass">)  [unwired: 7 in]
              }
              frame "Round" {
                n69 = Index Array(array=w218, index="Buoy to Round") -> (element=w217:T5)
                n70 = call "Initialize.vi"("Tolerance (m)"=w223, "Round side?"="Buoy Side", "Buoy to Round"=w217) -> ("RoundBuoys out"=w212:refnum<class "RoundBuoy.lvclass">)  [unwired: 7 in, 1 out]
                n71 = Flatten To String(anything=w212) -> (data string=w214:string)  [unwired: 3 in, 2 out]
                n72 = Bundle By Name(cluster=T47 {"OCU Command"=enum."Add Mission", "Data"=variant}, "Data"=w214) -> (w213:T47)
                n73 = call "Write.vi"("element"=w213, "NetworkStreamWriter in"=w221) -> ("NetworkStreamWriter out"=w222:refnum<class "NetworkStreamWriter.lvclass">)  [unwired: 8 in, 1 out]
              }
              frame "Pass" {
                # "build Pass Between Buoys mission"
                n74 = Index Array(array=w228, index #1="Starboard Buoy", index #2="Port Buoy") -> (element #1=w224:T5, element #2=w225:T5)
                n75 = call "Initialize.vi"("Buoy Pass 2"=w224, "Buoy Pass 1"=w225) -> ("PassBuoys out"=w230:refnum<class "PassBuoys.lvclass">)  [unwired: 8 in, 1 out]
                n76 = Flatten To String(anything=w230) -> (data string=w236:string)  [unwired: 3 in, 2 out]
                n77 = To Variant(anything=w236) -> (Variant=w237:variant)
                n78 = Bundle By Name(cluster=T47 {"OCU Command"=enum."Add Mission", "Data"=variant}, "Data"=w237) -> (w235:T47)
                n79 = To Variant(anything=w235) -> (Variant=w231:variant)
                n80 = call "Write.vi"("error in (no error)"=w229, "element"=w231, "NetworkStreamWriter in"=w234) -> ("error out"=w232:errorcluster, "NetworkStreamWriter out"=w233:refnum<class "NetworkStreamWriter.lvclass">)  [unwired: 7 in]
              }
              frame "Station" {
                # "user inputs two points as a line and we convert it to a square"
                n81 = Index Array(array=w246, index #1="Buoy A", index #2="Buoy B") -> (element #1=w243:T5, element #2=w242:T5)
                n82 = call "helper - UTM line to Square.vi"("Endpoint 2, UTM"=w242, "Endpoint 1, UTM"=w243) -> ("Endpoint 4, UTM"=w249:T5, "Endpoint 3, UTM"=w248:T5)
                n83 = call "Initialize.vi"("Duration (s)"=w239, "Buoy SE"=w242, "Buoy SW"=w243, "Buoy NE"=w249, "Buoy NW"=w248) -> ("StationKeeping out"=w250:refnum<class "StationKeeping.lvclass">)  [unwired: 5 in, 1 out]
                n84 = Flatten To String(anything=w250) -> (data string=w241:string)  [unwired: 3 in, 2 out]
                n85 = Bundle By Name(cluster=T47 {"OCU Command"=enum."Add Mission", "Data"=variant}, "Data"=w241) -> (w240:T47)
                n86 = call "Write.vi"("error in (no error)"=w247, "element"=w240, "NetworkStreamWriter in"=w251) -> ("error out"=w252:errorcluster, "NetworkStreamWriter out"=w253:refnum<class "NetworkStreamWriter.lvclass">)  [unwired: 7 in]
              }
            }
          }
        }
      }
      event "Boat to Point 0", "Boat to Point 1", "Boat to Point 2", "Boat to Point 3", "Boat to Point 4", "Local to Point 3", "Local to Point 2", "Local to Point 1", "Local to Point 0", "Local to Point 4": Value Change {
        # "save the current GPS location to one of the saved points."
        n87 = event-data() -> ()  [unwired: 1 in, 1 out]
        n88 = Build Array("Boat to Point 0", "Boat to Point 1", "Boat to Point 2", "Boat to Point 3", "Boat to Point 4") -> (w264:bool[])
        n89 = Build Array("Local to Point 0", "Local to Point 1", "Local to Point 2", "Local to Point 3", "Local to Point 4") -> (w255:bool[])
        n90 = for {
          tunnel: w264 -> [w277] mode=indexing
          i -> [w276]
          n91 = case shown="True" w277 {
            tunnel: w276 -> [_ w279]
            frame False {
            }
            frame True {
              # "load from boat GPS"
              n92 = local read "Stored Locations Array"() -> (w281:T5[])
              n93 = local read "Robot UTM Location"() -> (w278:T5)
              n94 = Replace Array Subset(array=w281, new element=w278, index=w279) -> (w280:T5[])
              n95 = local write "Stored Locations Array"(w280) -> ()
            }
          }
        }
        n96 = for {
          tunnel: w255 -> [w271] mode=indexing
          i -> [w270]
          n97 = case shown="True" w271 {
            tunnel: w270 -> [_ w272]
            frame False {
            }
            frame True {
              # "load from local GPS"
              n98 = local read "Stored Locations Array"() -> (w274:T5[])
              n99 = global read "2 Global.vi" "Robot UTM Location"() -> (w273:refnum<class "UTM_Location.lvclass">)
              n100 = Replace Array Subset(array=w274, new element=w273, index=w272) -> (w275:T5[])
              n101 = local write "Stored Locations Array"(w275) -> ()
            }
          }
        }
      }
      event "Update Constants": Value Change {
        # "To add a set of tuning constants, add a control constant in the cluster constant\nadd the control to the front panel and wire it into the bundler in the true case here; the  0x2 command\nreceive block will need to be edited as well as the TuningConstants global"
        n102 = event-data() -> ()  [unwired: 1 in, 1 out]
        n103 = case shown="True" "Update Constants" {
          tunnel: w285 -> [w289 w295]
          tunnel: w284 -> [w288 w294]
          tunnel: [w289 w293] -> w283
          tunnel: [w288 w292] -> w282
          frame False {
          }
          frame True {
            n104 = Bundle By Name(cluster=T47 {"OCU Command"=enum."Edit Control Values", "Data"=variant}, "Data"="Tuning Values") -> (w291:T47)
            n105 = call "Write.vi"("error in (no error)"=w294, "element"=w291, "NetworkStreamWriter in"=w295) -> ("error out"=w292:errorcluster, "NetworkStreamWriter out"=w293:refnum<class "NetworkStreamWriter.lvclass">)  [unwired: 7 in]
          }
        }
      }
      event "Log message": Key Up {
        # "Remove carriage\nreturn."
        # "Enter key?"
        n106 = event-data() -> ("ScanCode"=w298:i16)  [unwired: 1 in, 2 out]
        n107 = Equal?(x=w298, y=i16 28) -> (x = y?=w307:bool)
        n108 = Search and Replace String(replace all?=TRUE ("replace all? (F)"), input string="Log message", search string="\n" ("string"), replace string="") -> (result string=w304:string)  [unwired: 4 in, 3 out]
        n109 = case "Was the log message entered?" shown="True" w307 {
          tunnel: [w311 w320] -> w302
          tunnel: [w310 w319] -> w299
          tunnel: w301 -> [w310 w314]
          tunnel: w300 -> [w311 w318]
          tunnel: w304 -> [_ w315]
          frame False {
          }
          frame True {
            n110 = To Variant(anything=w315) -> (Variant=w322:variant)
            n111 = property on="Log message" class="Str"(error in=w314, "Value"="") -> (error out=w313:errorcluster)  [unwired: 1 in, 1 out]
            n112 = Bundle By Name(cluster=T47 {"OCU Command"=enum."Log Message", "Data"=variant}, "Data"=w322) -> (w321:T47)
            n113 = To Variant(anything=w321) -> (Variant=w316:variant)
            n114 = call "Write.vi"("error in (no error)"=w313, "element"=w316, "NetworkStreamWriter in"=w318) -> ("error out"=w319:errorcluster, "NetworkStreamWriter out"=w320:refnum<class "NetworkStreamWriter.lvclass">)  [unwired: 7 in]
          }
        }
      }
      event "Save Waypoints\nand PoI": Value Change {
        n115 = event-data() -> ()  [unwired: 1 in, 1 out]
        n116 = case "Save MDF" shown="True" "Save Waypoints\nand PoI" {
          frame False {
          }
          frame True {
            n117 = local read "Global No Sail Circles"() -> (w327:T35[])
            n118 = local read "Mission Object Array"() -> (w328:refnum<class "GenericMission.lvclass">[])
            n119 = call "0-Write MDF.vi"("Global No Sail Circles"=w327, "Missions (Object Array)"=w328) -> ()  [unwired: 3 in, 1 out]
          }
        }
      }
      event "Load MDF": Value Change {
        n120 = event-data() -> ()  [unwired: 1 in, 1 out]
        n121 = case "Load MDF" shown="True" "Load MDF" {
          tunnel: w332 -> [w335 w338]
          tunnel: [w335 w345] -> w331
          tunnel: w330 -> [w336 w340]
          tunnel: [w336 w343] -> w329
          frame False {
          }
          frame True {
            w342 = T47 {"OCU Command"=enum."Reset Missions/Waypts", "Data"=variant}  # clear missions
            n122 = To Variant(anything=w342) -> (Variant=w341:variant)
            n123 = call "Write.vi"("error in (no error)"=w338, "element"=w341, "NetworkStreamWriter in"=w340) -> ("error out"=w337:errorcluster, "NetworkStreamWriter out"=w339:refnum<class "NetworkStreamWriter.lvclass">)  [unwired: 7 in]
            n124 = call "0-Read MDF.vi"("Error in"=w337, "MDF file path"="Mission Def Filepath") -> ("Error out"=w347:errorcluster, "Global No Sail Circles"=w349:T35[], "Missions (Object Array)"=w348:refnum<class "GenericMission.lvclass">[])  [unwired: 1 in]
            n125 = for {
              tunnel: w348 -> [w360] mode=indexing
              shift-right: [w366] -> w346
              shift-left: w347 -> [w362]
              shift-right: [w364] -> w344
              shift-left: w339 -> [w365]
              n126 = Flatten To String(anything=w360, error in (no error)=w362) -> (data string=w361:string, error out=w363:errorcluster)  [unwired: 2 in, 1 out]
              n127 = To Variant(anything=w361) -> (Variant=w368:variant)
              n128 = Bundle By Name(cluster=T47 {"OCU Command"=enum."Add Mission", "Data"=variant}, "Data"=w368) -> (w369:T47)
              n129 = To Variant(anything=w369) -> (Variant=w367:variant)
              n130 = call "Write.vi"("error in (no error)"=w363, "element"=w367, "NetworkStreamWriter in"=w365) -> ("error out"=w366:errorcluster, "NetworkStreamWriter out"=w364:refnum<class "NetworkStreamWriter.lvclass">)  [unwired: 7 in]
            }
            n131 = local write "Mission Object Array"(w348) -> ()
            n132 = local write "Global No Sail Circles"(w349) -> ()
            n133 = for {
              tunnel: w349 -> [w352] mode=indexing
              shift-right: [w355] -> w345
              shift-left: w346 -> [w351]
              shift-right: [w353] -> w343
              shift-left: w344 -> [w354]
              n134 = To Variant(anything=w352) -> (Variant=w357:variant)
              n135 = Bundle By Name(cluster=T47 {"OCU Command"=enum."Add Global No-Sail", "Data"=variant}, "Data"=w357) -> (w358:T47)
              n136 = To Variant(anything=w358) -> (Variant=w356:variant)
              n137 = call "Write.vi"("error in (no error)"=w351, "element"=w356, "NetworkStreamWriter in"=w354) -> ("error out"=w355:errorcluster, "NetworkStreamWriter out"=w353:refnum<class "NetworkStreamWriter.lvclass">)  [unwired: 7 in]
            }
          }
        }
      }
      event "Reset Missions/Waypts": Value Change {
        n138 = event-data() -> ()  [unwired: 1 in, 1 out]
        n139 = case "Reset Missions" shown="True" "Reset Missions/Waypts" {
          tunnel: w374 -> [w378 w384]
          tunnel: w373 -> [w377 w383]
          tunnel: [w378 w382] -> w372
          tunnel: [w377 w381] -> w371
          frame False {
          }
          frame True {
            n140 = To Variant(anything=T47 {"OCU Command"=enum."Reset Missions/Waypts", "Data"=variant}) -> (Variant=w379:variant)
            n141 = call "Write.vi"("error in (no error)"=w383, "element"=w379, "NetworkStreamWriter in"=w384) -> ("error out"=w381:errorcluster, "NetworkStreamWriter out"=w382:refnum<class "NetworkStreamWriter.lvclass">)  [unwired: 7 in]
          }
        }
      }
      event "Mission Map": Mouse Up {
        # "add a waypoint to the list"
        n142 = event-data() -> ()  [unwired: 1 in, 1 out]
        n143 = case shown="\"Global No-Sail Zone\"" w387 {
          selector: w387 -> [_ _ w467 _ _]
          tunnel: w392 -> [w403 w429 w474 w492 w512]
          tunnel: [w401 w439 w471 w483 w503] -> w390
          tunnel: w391 -> [w402 w426 w456 w478 w510]
          tunnel: w386 -> [w396 _ w468 _ w493]
          tunnel: [w399 w437 w460 w486 w504] -> w389
          tunnel: w388 -> [w398 w436 w457 w487 w502]
          tunnel: w385 -> [_ _ _ _ w494]
          frame "Go to Waypoint", Default {
            n144 = property on="Mission Map" class="ImageControl"(error in=w403) -> (error out=w405:errorcluster, "Last Mouse Position"=w404:cluster{"X":i32, "Y":i32})  [unwired: 1 in, 1 out]
            n145 = call "Helper - Image To UTM.vi"("Image Descriptor"=w402, "Pixel Coordinates"=w404) -> ("UTM Location"=w394:T5)  [unwired: 1 in, 1 out]
            n146 = invoke on="Mission Map" class="ImageControl" method="Clear ROI"(error in=w405) -> (error out=w400:errorcluster)  [unwired: 2 in, 2 out]
            n147 = disable-structure shown="Enabled" {
              disable-tunnel: w396 -> [w412 w415]
              disable-tunnel: [w408 w419] -> w395
              disable-tunnel: w394 -> [w406 w414]
              frame Enabled {
                n148 = call "Initialize.vi"("Tolerance (m)"=w412, "Drive Location"=w406) -> ("Drive out"=w407:refnum<class "DriveTo.lvclass">)  [unwired: 8 in, 1 out]
                n149 = Flatten To String(anything=w407) -> (data string=w409:string)  [unwired: 3 in, 2 out]
                n150 = To Variant(anything=w409) -> (Variant=w410:variant)
                n151 = Bundle By Name(cluster=T47 {"OCU Command"=enum."Add Mission", "Data"=variant}, "Data"=w410) -> (w408:T47)
              }
              frame Disabled {
                n152 = call "init_waypoint.vi"("Coords"=w414, "Tolerance (m)"=w415) -> ("Waypoint Out"=w413:refnum<class "Waypoint.lvclass">)  [unwired: 9 in]
                n153 = Flatten To String(anything=w413) -> (data string=w416:string)  [unwired: 3 in, 2 out]
                n154 = To Variant(anything=w416) -> (Variant=w417:variant)
                n155 = Bundle By Name(cluster=T47 {"OCU Command"=enum."Set waypoint number", "Data"=variant}, "Data"=w417) -> (w419:T47)
              }
            }
            n156 = To Variant(anything=w395) -> (Variant=w397:variant)
            n157 = call "Write.vi"("error in (no error)"=w400, "element"=w397, "NetworkStreamWriter in"=w398) -> ("error out"=w401:errorcluster, "NetworkStreamWriter out"=w399:refnum<class "NetworkStreamWriter.lvclass">)  [unwired: 7 in]
          }
          frame "Global No-Sail Zone" {
            n158 = property on="Mission Map" class="ImageControl"(error in=w429) -> (error out=w428:errorcluster, "ROI"=w430:T51)  [unwired: 1 in, 1 out]
            n159 = call "helper- line ROI to 2 UTM Pts.vi"("ROI"=w430, "Image Descriptor"=w426) -> ("Endpoint UTM 2"=w425:T5, "Endpoint UTM 1"=w427:T5)
            n160 = Unbundle By Name(w425) -> ("East"=w423:dbl, "North"=w424:dbl)
            n161 = Unbundle By Name(w427) -> ("UTM Zone"=w431:dbl, "Hemisphere"=w432:enum16{"North", "South"}, "East"=w421:dbl, "North"=w422:dbl)
            n162 = call "2 XYPointsToDistanceAndAngle.vi"("East 2"=w424, "North 2"=w423, "East 1"=w422, "North 1"=w421) -> ("Distance"=w420:dbl)  [unwired: 6 in, 1 out]
            n163 = invoke on="Mission Map" class="ImageControl" method="Clear ROI"(error in=w428) -> (error out=w438:errorcluster)  [unwired: 2 in, 2 out]
            n164 = disable-structure shown="Enabled" {
              disable-tunnel: w420 -> [w445 w451]
              disable-tunnel: [w447 w455] -> w434
              disable-tunnel: T35 {"UTM Zone"=0.0, "Hemisphere"=enum."North", "East"=0.0, "North"=0.0, "Radius"=0.0} ("UTM Location") -> [w446 _]
              disable-tunnel: w422 -> [w444 _]
              disable-tunnel: w421 -> [w443 _]
              disable-tunnel: w432 -> [w442 _]
              disable-tunnel: w431 -> [w441 _]
              frame Enabled {
                n165 = Bundle By Name(cluster=w446, "UTM Zone"=w441, "Hemisphere"=w442, "East"=w443, "North"=w444, "Radius"=w445) -> (w440:T35)
                n166 = To Variant(anything=w440) -> (Variant=w448:variant)
                n167 = Bundle By Name(cluster=T47 {"OCU Command"=enum."Add Global No-Sail", "Data"=variant}, "Data"=w448) -> (w447:T47)
              }
              frame Disabled {
                n168 = call "init_waypoint.vi"("Tolerance (m)"=w451) -> ("Waypoint Out"=w450:refnum<class "Waypoint.lvclass">)  [unwired: 10 in]
                n169 = Flatten To String(anything=w450) -> (data string=w452:string)  [unwired: 3 in, 2 out]
                n170 = To Variant(anything=w452) -> (Variant=w453:variant)
                n171 = Bundle By Name(cluster=T47 {"OCU Command"=enum."Set waypoint number", "Data"=variant}, "Data"=w453) -> (w455:T47)
              }
            }
            n172 = To Variant(anything=w434) -> (Variant=w435:variant)
            n173 = call "Write.vi"("error in (no error)"=w438, "element"=w435, "NetworkStreamWriter in"=w436) -> ("error out"=w439:errorcluster, "NetworkStreamWriter out"=w437:refnum<class "NetworkStreamWriter.lvclass">)  [unwired: 7 in]
          }
          frame "Round Buoy Starboard", "Round Buoy Port" {
            n174 = property on="Mission Map" class="ImageControl"(error in=w474) -> (error out=w476:errorcluster, "Last Mouse Position"=w475:cluster{"X":i32, "Y":i32})  [unwired: 1 in, 1 out]
            n175 = Equal?(x=w467, y=Mission_Type_Radio_Buttons."Round Buoy Port" ("Mission Type 2")) -> (x = y?=w462:bool)
            n176 = call "Helper - Image To UTM.vi"("Image Descriptor"=w456, "Pixel Coordinates"=w475) -> ("UTM Location"=w469:T5)  [unwired: 1 in, 1 out]
            n177 = invoke on="Mission Map" class="ImageControl" method="Clear ROI"(error in=w476) -> (error out=w471:errorcluster)  [unwired: 2 in, 2 out]
            n178 = Select(t=enum16{"Starboard", "Port"}."Port" ("Round side?"), s=w462, f=enum16{"Starboard", "Port"}."Starboard" ("Round side?")) -> (s? t:f=w463:enum16{"Starboard", "Port"})
            n179 = call "Initialize.vi"("Tolerance (m)"=w468, "Round side?"=w463, "Buoy to Round"=w469) -> ("RoundBuoys out"=w461:refnum<class "RoundBuoy.lvclass">)  [unwired: 7 in, 1 out]
            n180 = Flatten To String(anything=w461) -> (data string=w470:string)  [unwired: 3 in, 2 out]
            n181 = To Variant(anything=w470) -> (Variant=w472:variant)
            n182 = Bundle By Name(cluster=T47 {"OCU Command"=enum."Add Mission", "Data"=variant}, "Data"=w472) -> (w458:T47)
            n183 = To Variant(anything=w458) -> (Variant=w459:variant)
            n184 = call "Write.vi"("element"=w459, "NetworkStreamWriter in"=w457) -> ("NetworkStreamWriter out"=w460:refnum<class "NetworkStreamWriter.lvclass">)  [unwired: 8 in, 1 out]
          }
          frame "Pass Between Buoys" {
            # "build Pass Between Buoys mission"
            n185 = property on="Mission Map" class="ImageControl"(error in=w492) -> (error out=w484:errorcluster, "ROI"=w477:T51)  [unwired: 1 in, 1 out]
            n186 = invoke on="Mission Map" class="ImageControl" method="Clear ROI"(error in=w484) -> (error out=w485:errorcluster)  [unwired: 2 in, 2 out]
            n187 = call "helper- line ROI to 2 UTM Pts.vi"("ROI"=w477, "Image Descriptor"=w478) -> ("Endpoint UTM 2"=w480:T5, "Endpoint UTM 1"=w479:T5)
            n188 = call "Initialize.vi"("Buoy Pass 2"=w480, "Buoy Pass 1"=w479) -> ("PassBuoys out"=w481:refnum<class "PassBuoys.lvclass">)  [unwired: 8 in, 1 out]
            n189 = Flatten To String(anything=w481) -> (data string=w489:string)  [unwired: 3 in, 2 out]
            n190 = To Variant(anything=w489) -> (Variant=w490:variant)
            n191 = Bundle By Name(cluster=T47 {"OCU Command"=enum."Add Mission", "Data"=variant}, "Data"=w490) -> (w488:T47)
            n192 = To Variant(anything=w488) -> (Variant=w482:variant)
            n193 = call "Write.vi"("error in (no error)"=w485, "element"=w482, "NetworkStreamWriter in"=w487) -> ("error out"=w483:errorcluster, "NetworkStreamWriter out"=w486:refnum<class "NetworkStreamWriter.lvclass">)  [unwired: 7 in]
          }
          frame "Station Keeping" {
            # "user inputs two points as a line and we convert it to a square"
            n194 = property on="Mission Map" class="ImageControl"(error in=w512) -> (error out=w500:errorcluster, "ROI"=w511:T51)  [unwired: 1 in, 1 out]
            n195 = call "helper- line ROI to 2 UTM Pts.vi"("ROI"=w511, "Image Descriptor"=w510) -> ("Endpoint UTM 2"=w495:T5, "Endpoint UTM 1"=w496:T5)
            n196 = call "helper - UTM line to Square.vi"("Endpoint 2, UTM"=w495, "Endpoint 1, UTM"=w496) -> ("Endpoint 4, UTM"=w498:T5, "Endpoint 3, UTM"=w497:T5)
            n197 = invoke on="Mission Map" class="ImageControl" method="Clear ROI"(error in=w500) -> (error out=w501:errorcluster)  [unwired: 2 in, 2 out]
            n198 = call "Initialize.vi"("Tolerance (m)"=w493, "Duration (s)"=w494, "Buoy SE"=w495, "Buoy SW"=w496, "Buoy NE"=w498, "Buoy NW"=w497) -> ("StationKeeping out"=w499:refnum<class "StationKeeping.lvclass">)  [unwired: 4 in, 1 out]
            n199 = Flatten To String(anything=w499) -> (data string=w507:string)  [unwired: 3 in, 2 out]
            n200 = To Variant(anything=w507) -> (Variant=w508:variant)
            n201 = Bundle By Name(cluster=T47 {"OCU Command"=enum."Add Mission", "Data"=variant}, "Data"=w508) -> (w506:T47)
            n202 = To Variant(anything=w506) -> (Variant=w505:variant)
            n203 = call "Write.vi"("error in (no error)"=w501, "element"=w505, "NetworkStreamWriter in"=w502) -> ("error out"=w503:errorcluster, "NetworkStreamWriter out"=w504:refnum<class "NetworkStreamWriter.lvclass">)  [unwired: 7 in]
          }
        }
      }
      event Value Change {
        # "gray out the appropriate numeric controls"
        # "set input tool"
        # "Adjust OCU controls for the correct mission input style"
        n204 = event-data() -> ("NewVal"=w518:T15)  [unwired: 1 in]
        n205 = case shown="\"Station Keeping\"" w518 {
          tunnel: [T49."Enabled" ("Disabled") w522 T49."Enabled" ("Disabled")] -> w517
          tunnel: [T49."Disabled and Grayed Out" ("Disabled") w522 T49."Enabled" ("Disabled")] -> w516
          frame "Go to Waypoint", Default {
          }
          frame "Pass Between Buoys", "Global No-Sail Zone" {
            w522 = T49."Disabled and Grayed Out" ("Disabled")
            # "\"Pass Between Buoys\"\nhas neither input"
          }
          frame "Station Keeping" {
          }
        }
        n206 = case shown="\"Pass Between Buoys\", \"Global No-Sail Zone\"" w518 {
          tunnel: [w525 w526 w527] -> w519
          frame "Go to Waypoint", Default {
            w525 = u32 1 items=["Zoom Tool"=8, "Selection Tool"=0, "Pan Tool"=9, "Point Tool"=1, "Line Tool"=2, "Rectangle Tool"=3, "Rotated Rectangle Tool"=12, "Polyline Tool"=10, "Polygon Tool"=5, "Freehand Tool"=11, "Closed Freehand Tool"=6, "Ellipse Tool"=4, "Annulus Tool"=7] ("Current ROI Tool")
          }
          frame "Station Keeping" {
            w526 = u32 2 items=["Zoom Tool"=8, "Selection Tool"=0, "Pan Tool"=9, "Point Tool"=1, "Line Tool"=2, "Rectangle Tool"=3, "Rotated Rectangle Tool"=12, "Polyline Tool"=10, "Polygon Tool"=5, "Freehand Tool"=11, "Closed Freehand Tool"=6, "Ellipse Tool"=4, "Annulus Tool"=7] ("Current ROI Tool")
          }
          frame "Pass Between Buoys", "Global No-Sail Zone" {
            w527 = u32 2 items=["Zoom Tool"=8, "Selection Tool"=0, "Pan Tool"=9, "Point Tool"=1, "Line Tool"=2, "Rectangle Tool"=3, "Rotated Rectangle Tool"=12, "Polyline Tool"=10, "Polygon Tool"=5, "Freehand Tool"=11, "Closed Freehand Tool"=6, "Ellipse Tool"=4, "Annulus Tool"=7] ("Current ROI Tool")
          }
        }
        n207 = property on="Tolerance" class="DigNum (strict)"("DisabledEnum"=w517) -> ()  [unwired: 2 in, 2 out]
        n208 = property on="Time(s)" class="DigNum (strict)"("DisabledEnum"=w516) -> ()  [unwired: 2 in, 2 out]
        n209 = property on="Mission Map" class="ImageControl"("Current ROI Tool"=w519) -> ()  [unwired: 2 in, 2 out]
      }
    }
    n210 = local read "Setpoints to boat"() -> (w94:T28)
    n211 = local read "OVERRIDE RUDDER?"() -> (w100:bool)
    n212 = local read "OVERRIDE SAIL?"() -> (w95:bool)
    n213 = Unbundle By Name(w102) -> ("Sail Position"=w97:T29, "Rudder Angle"=w98:T30)
    n214 = Unbundle By Name(w94) -> ("Sail Position"=w93:T29, "Rudder Angle"=w92:T30)
    n215 = call "eStopShared.vi"("Command"=eStopCommand."Set E-Stop", "E-Stop"="Stop") -> ("E-Stop Out"=w107:bool)  [unwired: 8 in, 1 out]
    n216 = Select(t=w97, s=w95, f=w93) -> (s? t:f=→"Sail Position":T29)
    n217 = Select(t=w98, s=w100, f=w92) -> (s? t:f=→"Rudder Position":T30)
  }
  n218 = while {
    stop <- w537 stop-if-true
    n219 = global read "2 Global.vi" "Sensor Status"() -> (w535:T1)
    "Sensor Status" <- w535
    n220 = Unbundle By Name(w535) -> ("Sensor OK"=w531:T2, "Sensor Initialized"=w530:T2, "GPS Lock"=w528:T2)
    n221 = And(x=w531, y=w530) -> (x .and. y?=w529:T2)
    n222 = case shown="True" "Enable \nLocal GPS" {
      tunnel: w529 -> [_ w540]
      frame False {
        n223 = Wait Until Next ms Multiple(millisecond multiple=u32 100) -> ()  [unwired: 1 out]
      }
      frame True {
        n224 = case shown="False" w540 {
          tunnel: [w547 w549] -> w544
          tunnel: "GPS COM port" -> [w548 w549]
          tunnel: [w546 _] -> w542
          frame False {
            n225 = call "1A Helper - Init Sensor.vi"("VISA Refnum in"=w548) -> ("error out"=w546:errorcluster, "VISA Refnum out"=w547:refnum<visa-resource-name>)  [unwired: 8 in, 1 out]
          }
          frame True {
          }
        }
        n226 = call "1A Read Sensor Data.vi"("error (in)"=w542, "VISA resource name (in)"=w544) -> ("error (out)"=w541:errorcluster)  [unwired: 8 in, 1 out]
        n227 = case shown="Error" w541 {
          frame No Error {
          }
          frame Error {
            n228 = local write "Enable \nLocal GPS"(FALSE ("Enable \nLocal GPS")) -> ()
          }
        }
      }
    }
    n229 = call "eStopShared.vi"("Command"=eStopCommand."Get E-Stop") -> ("E-Stop Out"=w537:bool)  [unwired: 9 in, 1 out]
    n230 = Select(t=T49."Enabled" ("Disabled"), s=w528, f=T49."Disabled and Grayed Out" ("Disabled")) -> (s? t:f=w532:T49)
    n231 = property on="Local to Point 0" class="Bool"("DisabledEnum"=w532) -> ()  [unwired: 2 in, 2 out]
    n232 = property on="Local to Point 1" class="Bool"("DisabledEnum"=w532) -> ()  [unwired: 2 in, 2 out]
    n233 = property on="Local to Point 2" class="Bool"("DisabledEnum"=w532) -> ()  [unwired: 2 in, 2 out]
    n234 = property on="Local to Point 3" class="Bool"("DisabledEnum"=w532) -> ()  [unwired: 2 in, 2 out]
    n235 = property on="Local to Point 4" class="Bool"("DisabledEnum"=w532) -> ()  [unwired: 2 in, 2 out]
  }
  n236 = call "Close.vi"("error in (no error)"=w24, "NetworkStreamReader in"=w25) -> ()  [unwired: 9 in, 1 out]
  n237 = call "Close.vi"("error in (no error)"=w18, "NetworkStreamWriter in"=w19) -> ()  [unwired: 9 in, 1 out]
